vi "Write Configuration.vi"(8 "error in (no error)":errorcluster, 10 "Configuration":refnum<class "Configuration.lvclass">, 11 "Control Box in":refnum<class "Control Box.lvclass">) -> (0 "error out":errorcluster, 3 "Control Box out":refnum<class "Control Box.lvclass">)   [LabVIEW 2018, in "Control Box.lvlib" / "Control Box.lvclass"]
uses:
  Control Box.lvclass
  builds/Configuration.lvlibp/Configuration.lvclass
  Control Box.lvclass/Control Box.ctl
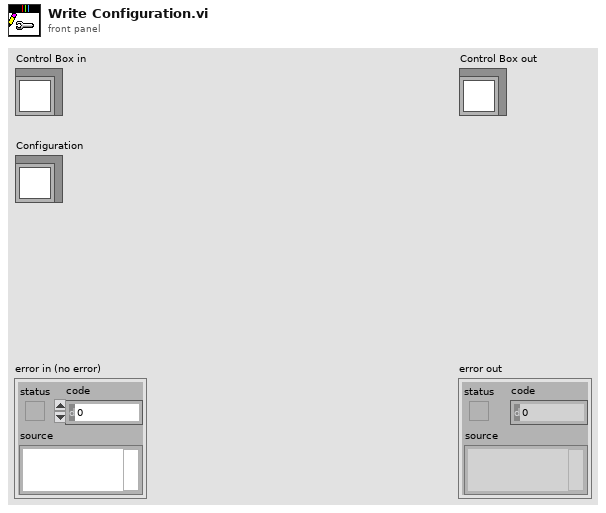
[diagram p1: front panel]
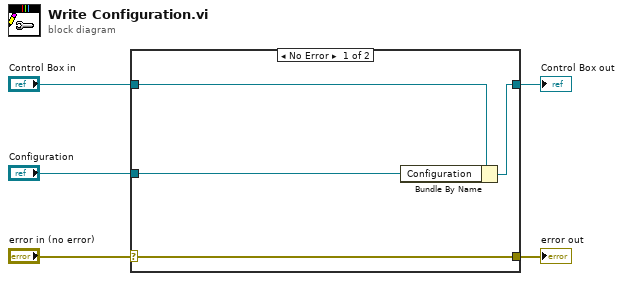
[diagram p0: block diagram]
diagram:
  n1 = case shown="No Error" "error in (no error)" {
    selector: "error in (no error)" -> [w9 w10]
    tunnel: [w9 w10] -> w4
    tunnel: [w7 w11] -> w2
    tunnel: "Control Box in" -> [w8 w11]
    tunnel: "Configuration" -> [w6 _]
    frame No Error {
      n2 = Bundle By Name(cluster=w8, "Configuration"=w6) -> (w7:refnum<class "Control Box.lvclass">)
    }
    frame Error {
    }
  }
  "error out" <- w4
  "Control Box out" <- w2
